vi "Update Tree Items.vi"(7 "Item":string, 9 "Status":T1=enum."Passed", 10 "Child Text":string, 11 "Test Tree In":refnum<class "Test Tree.lvclass">) -> (3 "Test Tree Out":refnum<class "Test Tree.lvclass">)   [LabVIEW 2020, in "Test Tree.lvclass"]
uses:
  Test Tree.lvclass
  Result/Status.ctl
  Test Tree.lvclass/Test Tree.ctl
  Utilities/LUnit Utilities.lvlib
  Result/Result.lvlib
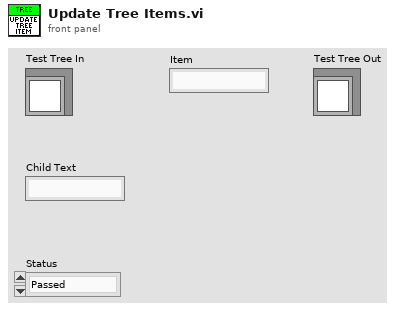
[diagram p1: front panel]
types:
  T1 = typedef "Result.lvlib/Status.ctl" = enum16{"", "Passed", "Failed", "Error", "Skipped", "Setup Error", "Broken", "Teardown Error"}
  T2 = map{string, cluster{"Left Cell String":string, "Child Text":string[], "Item Indent":i32, "Child Only?":bool, "Glyph Index":i32}}
  T3 = cluster{"Left Cell String":string, "Child Text":string[], "Item Indent":i32, "Child Only?":bool, "Glyph Index":i32}
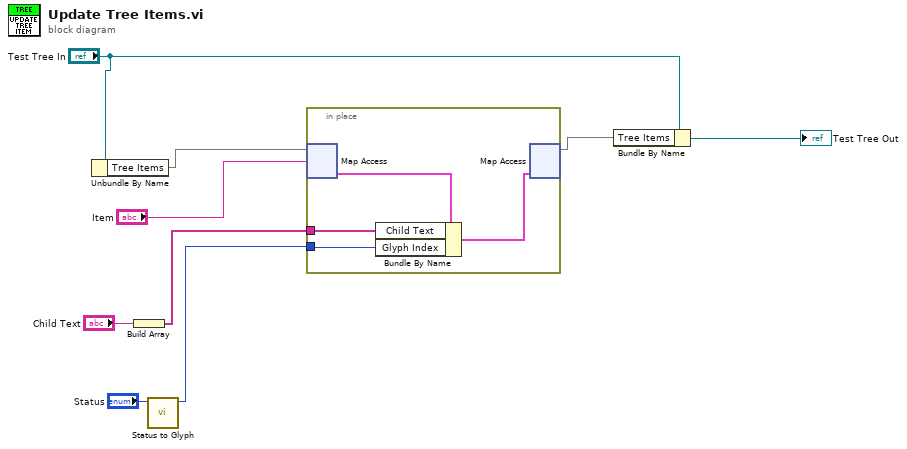
[diagram p0: block diagram]
diagram:
  n1 = Unbundle By Name("Test Tree In") -> ("Tree Items"=w7:T2)
  n2 = Build Array("Child Text") -> (w3:string[])
  n3 = call "Status to Glyph.vi"("Status"="Status") -> ("Listbox Symbol Ring Constant"=w1:i32)  [unwired: 10 in]
  n4 = in-place {
    in-place-border: w3 -> [w11]
    in-place-border: w1 -> [w10]
    n5 = in-place-map #1(w7, "Item") -> (w13:T3)  [unwired: 1 in, 1 out]
    n6 = Bundle By Name(cluster=w13, "Child Text"=w11, "Glyph Index"=w10) -> (w12:T3)
    n7 = in-place-map #1(w12) -> (w6:T2)  [unwired: 1 in, 2 out]
  }
  n8 = Bundle By Name(cluster="Test Tree In", "Tree Items"=w6) -> (→"Test Tree Out":refnum<class "Test Tree.lvclass">)
